vi "Read Nested Viewable Enqueuers.vi"(10 "Popup ViewManager in":refnum<class "Popup ViewManager.lvclass">) -> (1 "Viewable Names":string[](array[string]), 2 "Nested Enqueuers":refnum<class "Message Enqueuer.lvclass">[](array[class]))   [LabVIEW 2019, in "Popup ViewManager.lvlib" / "Popup ViewManager.lvclass"]
uses:
  <vilib>/gpm_packages/@cs/popup-viewmanager/Source/Popup ViewManager/Popup ViewManager.lvclass
  <vilib>/ActorFramework/Message Enqueuer/Message Enqueuer.lvclass
  <vilib>/gpm_packages/@cs/popup-viewmanager/Source/Popup ViewManager/Popup ViewManager.lvclass/Popup ViewManager.ctl
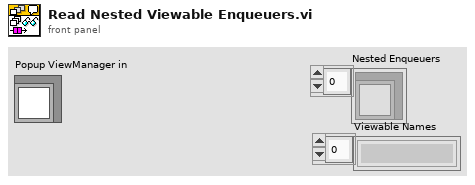
[diagram p1: front panel]
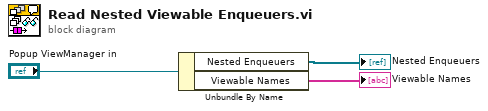
[diagram p0: block diagram]
diagram:
  n1 = Unbundle By Name("Popup ViewManager in") -> ("Nested Enqueuers"=→"Nested Enqueuers":refnum<class "Message Enqueuer.lvclass">[], "Viewable Names"=→"Viewable Names":string[])
